vi "Check GB and Edge Proximity.vi"(8 "Border Radius":dbl=3.0, 9 "Grain Boundary Location":dbl=3.0, 10 "Lattice Vectors":dbl[][](array[numeric])=[[10.1, 0.0, 0.0]], 11 "Atom (Cartesian)":dbl[](array[numeric])=[10.1, 0.0, 0.0]) -> (2 "Along GB?":bool, 3 "Along Border?":bool)   [LabVIEW 2010]
panel:
  # "a"
  # "b"
  # "c"
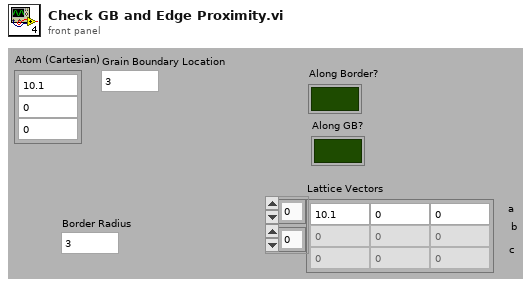
[diagram p1: front panel]
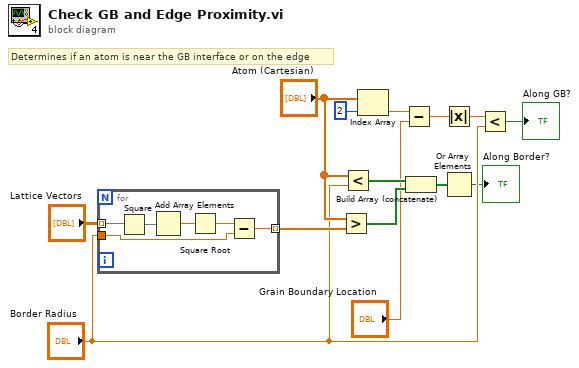
[diagram p0: block diagram]
diagram:
  # "Determines if an atom is near the GB interface or on the edge"
  n1 = for {
    tunnel: "Lattice Vectors" -> [w16] mode=indexing
    tunnel: "Border Radius" -> [w20]
    tunnel: [w19] -> w12 mode=indexing
    n2 = Square(x=w16) -> (x^2=w18:dbl[])
    n3 = Add Array Elements(numeric array=w18) -> (sum=w17:dbl)
    n4 = Square Root(x=w17) -> (sqrt(x)=w15:dbl)
    n5 = Subtract(x=w15, y=w20) -> (x-y=w19:dbl)
  }
  n6 = Greater?(x="Atom (Cartesian)", y=w12) -> (0:w11:bool[])
  n7 = Less?(x="Atom (Cartesian)", y="Border Radius") -> (x < y?=w14:bool[])
  n8 = Index Array(array="Atom (Cartesian)", index=2) -> (element=w8:dbl)
  n9 = Subtract(x=w8, y="Grain Boundary Location") -> (x-y=w6:dbl)
  n10 = Build Array (concatenate)(w14, w11) -> (w13:bool[])
  n11 = Absolute Value(x=w6) -> (abs(x)=w5:dbl)
  n12 = Or Array Elements(Boolean array=w13) -> (logical OR=→"Along Border?":bool)
  n13 = Less?(x=w5, y="Border Radius") -> (x < y?=→"Along GB?":bool)
